vi "Dual Camera Delay Capture.vi"(7 "Calling VI Ref":refnum<vi>) -> ()   [LabVIEW 2016]
uses:
  Dual Camera Control Type Defs/Dual Camera Notifier Type.ctl
  Dual Camera Control Type Defs/Dual Camera Actions.ctl
  <vilib>/Utility/miscctls.llb/LVPointTypeDef.ctl
  Dual Camera Control Type Defs/Dual Camera Delay Capture Actions.ctl
panel:
  in  "Capture":bool
  out "Current Cycle":u32=1
  out "Current Delay Time (s)":dbl=1.0 format="%.1f"
  in  "Quit":bool
  in  "Cycle Delay (s)":u32
  in  "Number of Cycles":u32=1
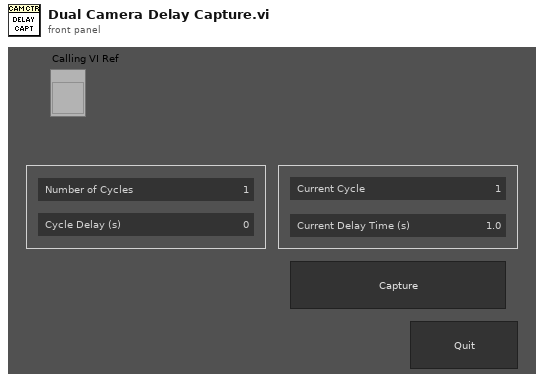
[diagram p1: front panel]
types:
  T1 = typedef "Dual Camera Delay Capture Actions.ctl" = enum16{"Idle", "Start Acquisition", "Get Images", "Check Cycle", "Delay", "Abort", "Exit Loop", "Quit"}
  T2 = enum16{"Always On", "Always Off", "Off While Running"}
  T3 = typedef "LVPointTypeDef.ctl" = cluster{"Horizontal":i16, "Vertical":i16}
  T4 = typedef "Dual Camera Notifier Type.ctl" = cluster{"Actions":T5, "Exposure Time (s)":dbl, "Num of Frames":u32, "Save Path":path, "Running?":bool, "Active Cameras":bool[]}
  T5 = typedef "Dual Camera Actions.ctl" = enum16{"Idle", "Exposure Time", "Preview", "Capture", "Set Save Path", "Lasers On", "Lasers Off", "Start Acquisition", "Abort", "Exit Loop", "Quit"}
  T6 = typedef "LVRectTypeDef.ctl" = cluster{"Left":i16, "Top":i16, "Right":i16, "Bottom":i16}
  T7 = typedef "LVBoundsTypeDef.ctl" = cluster{"Width":u32, "Height":u32}
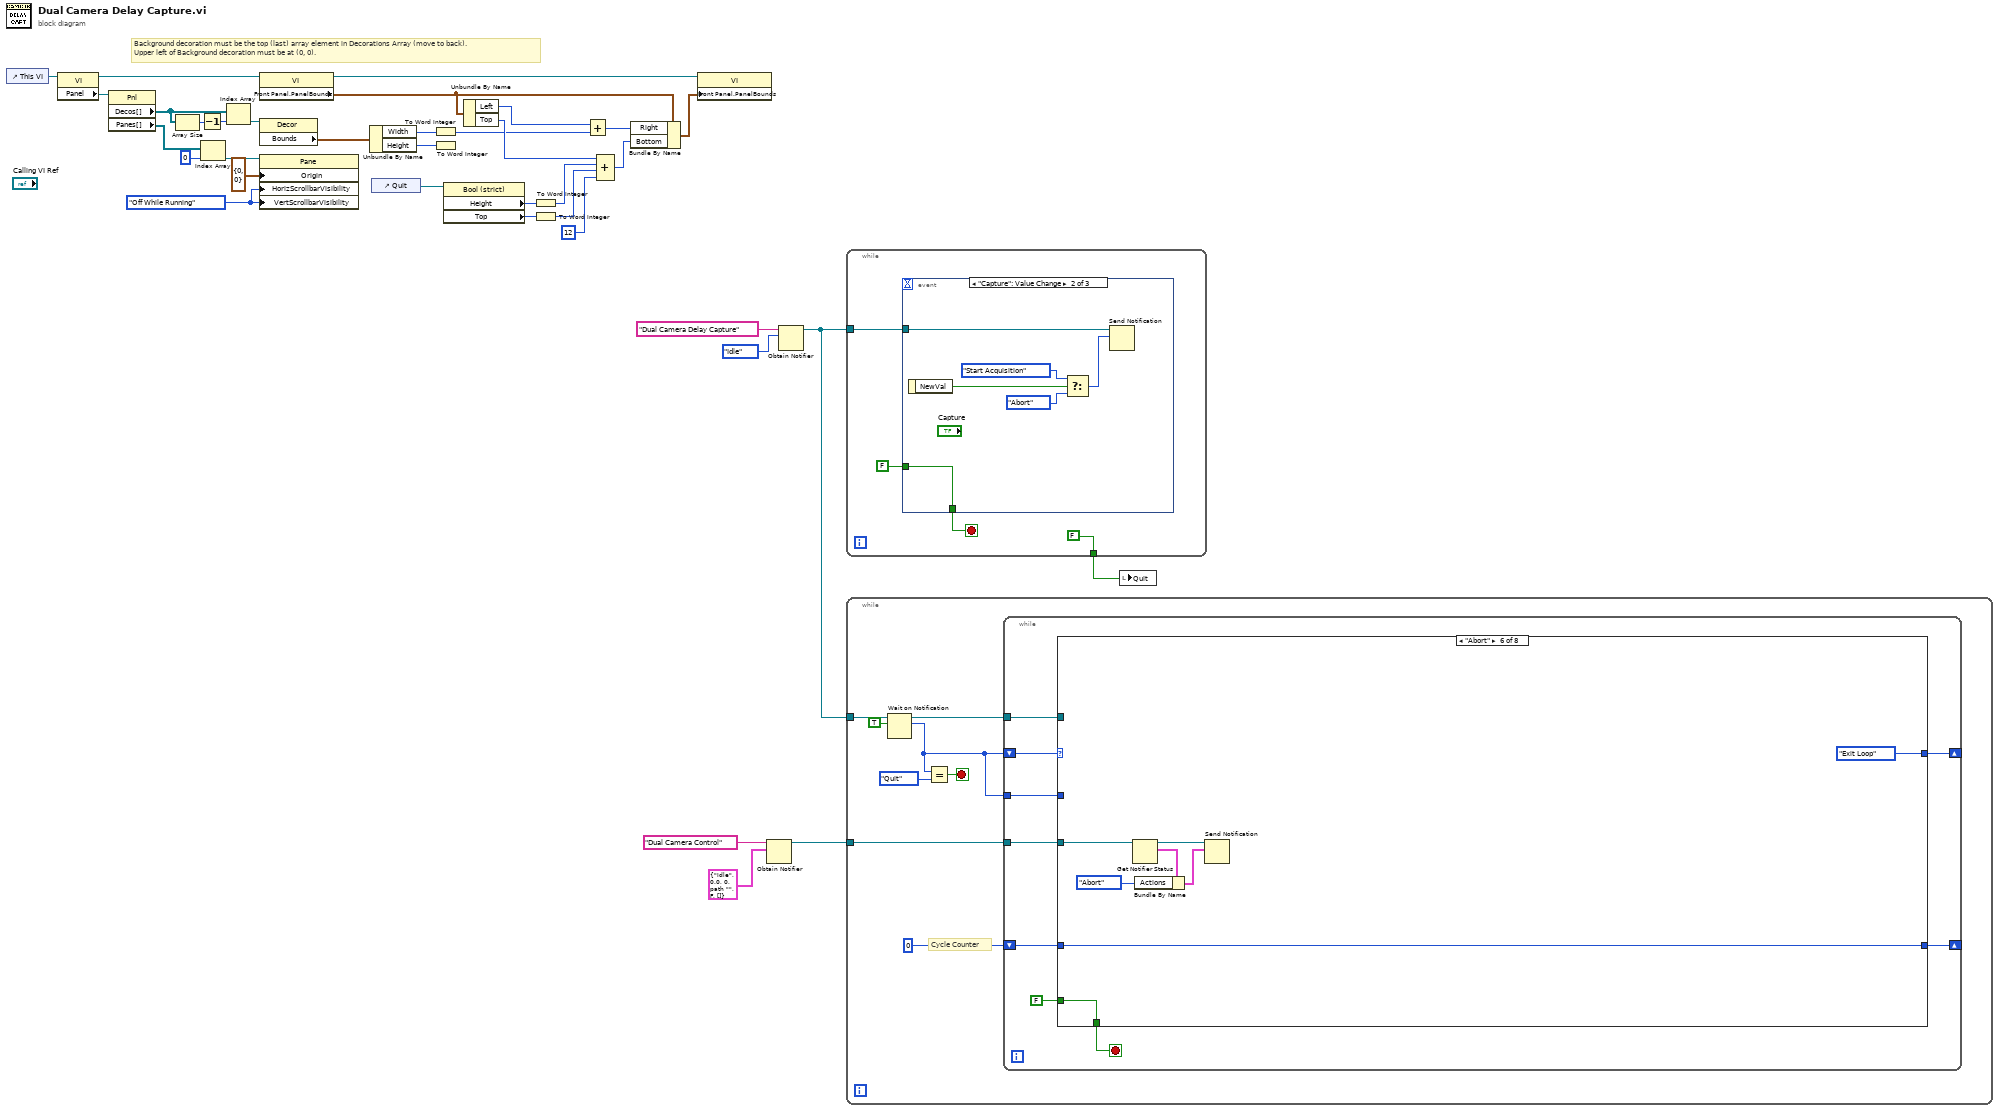
[diagram p0: block diagram]
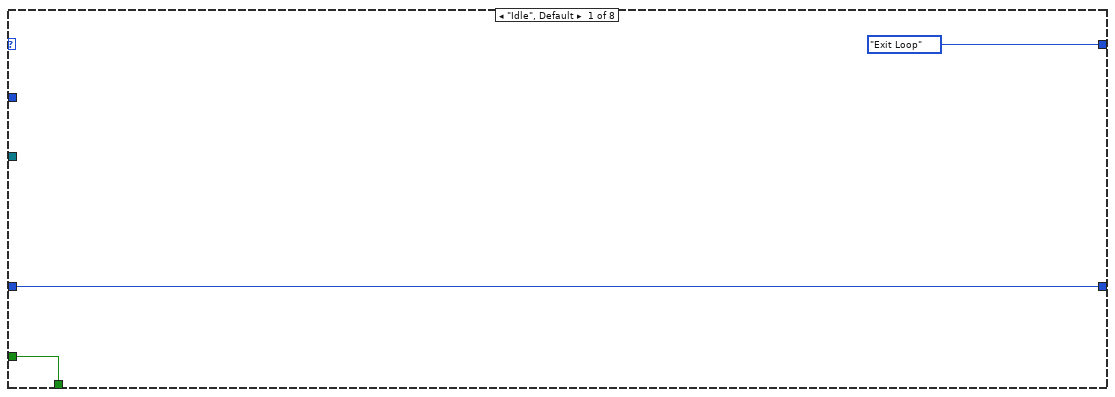
[diagram p2: hidden frame]
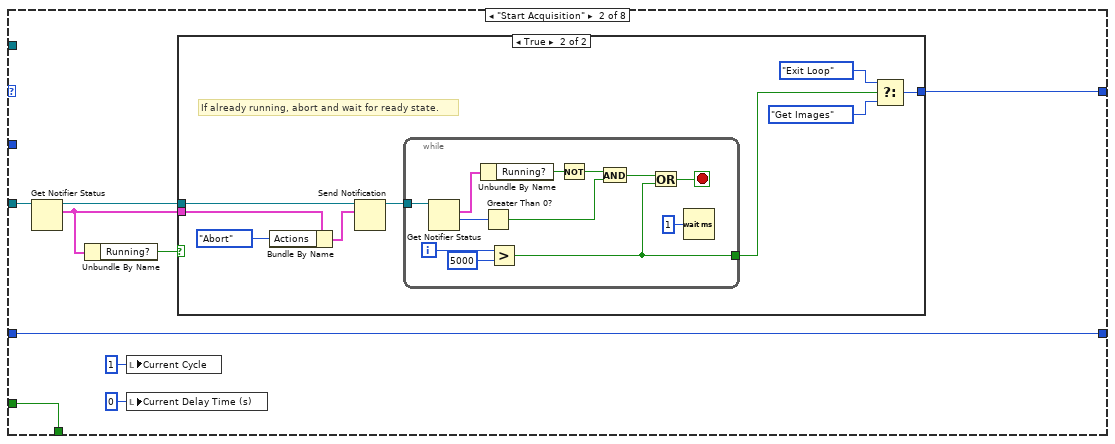
[diagram p3: hidden frame]
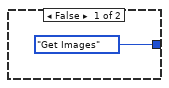
[diagram p4: hidden frame]
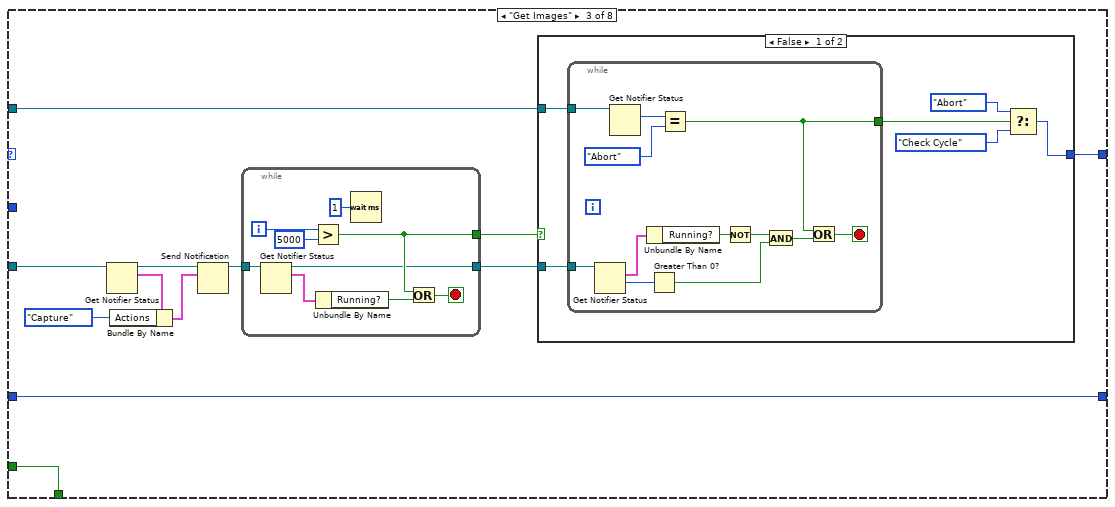
[diagram p5: hidden frame]
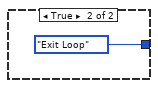
[diagram p6: hidden frame]
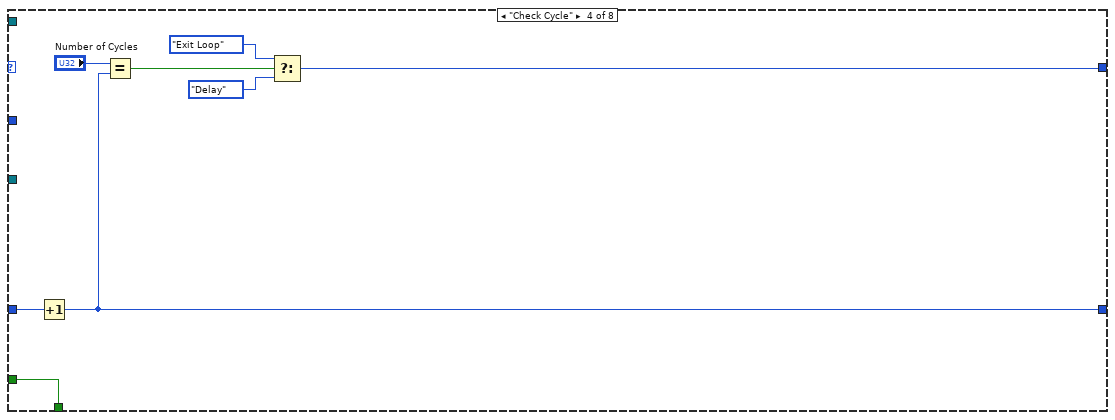
[diagram p7: hidden frame]
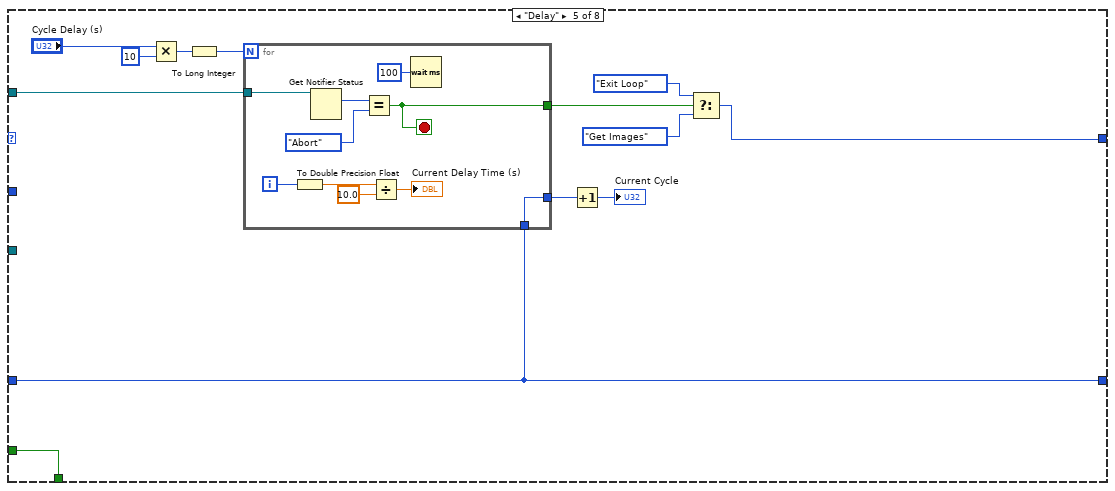
[diagram p8: hidden frame]
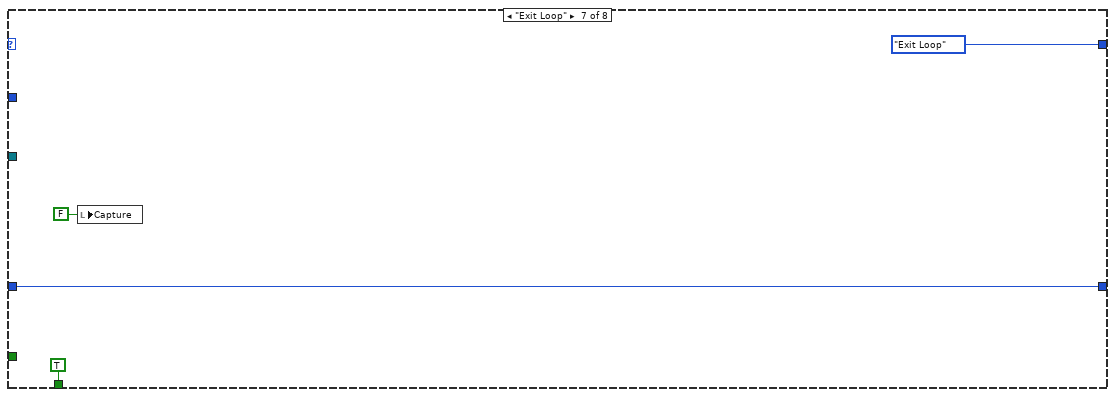
[diagram p9: hidden frame]
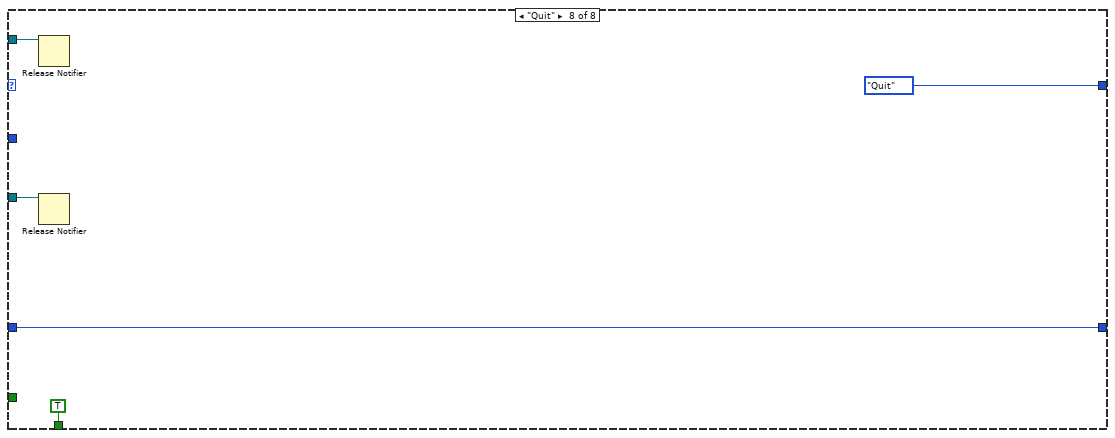
[diagram p10: hidden frame]
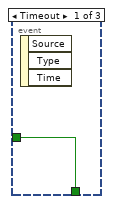
[diagram p11: hidden frame]
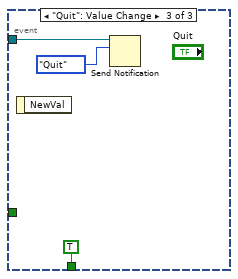
[diagram p12: hidden frame]
diagram:
  w17 = T2."Off While Running" ("Vertical Scrollbar Visibility")
  # "Background decoration must be the top (last) array element in Decorations Array (move to back).\nUpper left of Background decoration must be at (0, 0)."
  n1 = control-ref of="This VI"() -> (w9:refnum<vi>)
  n2 = property class="VI"(reference=w9) -> (reference out=w18:refnum<vi>, "Panel"=w10:refnum<vi>)  [unwired: 1 in, 1 out]
  n3 = property class="Pnl"(reference=w10) -> ("Decos[]"=w8:refnum<vi>[], "Panes[]"=w14:refnum<vi>[])  [unwired: 1 in, 2 out]
  n4 = Array Size(array=w8) -> (size(s)=w6:i32)
  n5 = Decrement(x=w6) -> (x-1=w7:i32)
  n6 = Index Array(array=w14, index=0) -> (element=w13:refnum<vi>)
  n7 = Index Array(array=w8, index=w7) -> (element=w16:refnum<vi>)
  n8 = property class="VI"(reference=w18) -> (reference out=w20:refnum<vi>, "Front Panel.PanelBounds"=w21:T6)  [unwired: 1 in, 1 out]
  n9 = property class="Decor"(reference=w16) -> ("Bounds"=w19:T7)  [unwired: 1 in, 2 out]
  n10 = property class="Pane"(reference=w13, "Origin"=T3 {"Horizontal"=0, "Vertical"=0}, "HorizScrollbarVisibility"=w17, "VertScrollbarVisibility"=w17) -> ()  [unwired: 1 in, 2 out]
  n11 = Unbundle By Name(w19) -> ("Width"=w24:u32, "Height"=w27:u32)
  n12 = control-ref of="Quit"() -> (w11:refnum<vi>)
  n13 = To Word Integer(number=w24) -> (16bit integer=w26:i16)
  n14 = To Word Integer(number=w27) -> ()  [unwired: 1 out]
  n15 = property class="Bool (strict)"(reference=w11) -> ("Height"=w29:u32, "Top"=w30:i32)  [unwired: 1 in, 2 out]
  n16 = Unbundle By Name(w21) -> ("Left"=w23:i16, "Top"=w34:i16)
  n17 = To Word Integer(number=w29) -> (16bit integer=w32:i16)
  n18 = To Word Integer(number=w30) -> (16bit integer=w33:i16)
  n19 = Add(x=w23, y=w26) -> (x+y=w25:i16)
  n20 = Compound Arithmetic op=ADD(w34, w32, w33, i16 12 ("y")) -> (w28:i16)
  n21 = Bundle By Name(cluster=w21, "Right"=w25, "Bottom"=w28) -> (w22:T6)
  n22 = property class="VI"(reference=w20, "Front Panel.PanelBounds"=w22) -> ()  [unwired: 1 in, 2 out]
  n23 = Obtain Notifier(name (unnamed)="Dual Camera Control", notification data type=T4 {"Actions"=enum."Idle", "Exposure Time (s)"=0.0, "Num of Frames"=0, "Save Path"=path "", "Running?"=FALSE, "Active Cameras"=[]} ("Dual Camera Notifier Type")) -> (notifier out=w4:refnum<notifier>)  [unwired: 2 in, 2 out]
  n24 = Obtain Notifier(name (unnamed)="Dual Camera Delay Capture", notification data type=Dual_Camera_Delay_Capture_Actions."Idle" ("Actions")) -> (notifier out=w1:refnum<notifier>)  [unwired: 2 in, 2 out]
  n25 = while {
    tunnel: [FALSE] -> w35
    tunnel: w1 -> [w37]
    stop <- w39 stop-if-true
    n26 = event shown="[1] \"Capture\": Value Change" {
      selector: _ -> [_ _ _]
      dyn-events: _ -> [_ _ _]
      timeout: _ -> [_ _ _]
      tunnel: FALSE -> [w41 w47 _]
      tunnel: [w41 w47 TRUE] -> w39
      tunnel: w37 -> [_ w43 w49]
      event Timeout {
        n27 = event-data() -> ()  [unwired: 1 in, 3 out]
      }
      event "Capture": Value Change {
        n28 = event-data() -> ("NewVal"=w46:bool)  [unwired: 1 in]
        n29 = Select(t=Dual_Camera_Delay_Capture_Actions."Start Acquisition" ("notification"), s=w46, f=Dual_Camera_Delay_Capture_Actions."Abort" ("notification")) -> (s? t:f=w42:T1)
        n30 = Send Notification(notification=w42, notifier=w43) -> ()  [unwired: 1 in, 2 out]
      }
      event "Quit": Value Change {
        n31 = event-data() -> ()  [unwired: 1 in, 1 out]
        n32 = Send Notification(notification=Dual_Camera_Delay_Capture_Actions."Quit", notifier=w49) -> ()  [unwired: 1 in, 2 out]
      }
    }
  }
  n33 = while {
    tunnel: w1 -> [w58]
    tunnel: w4 -> [w54]
    stop <- w56 stop-if-true
    # "Cycle Counter"
    n34 = Wait on Notification(notifier=w58, ignore previous (F)=TRUE) -> (notifier out=w55:refnum<notifier>, notification=w53:T1)  [unwired: 2 in, 2 out]
    n35 = Equal?(x=w53, y=Dual_Camera_Delay_Capture_Actions."Quit") -> (x = y?=w56:bool)
    n36 = while {
      shift-right: [w61] -> _
      shift-left: w53 -> [w66]
      tunnel: w55 -> [w67]
      tunnel: w53 -> [w63]
      tunnel: w54 -> [w62]
      shift-right: [w59] -> _
      shift-left: u32 0 -> [w60]
      stop <- w64 stop-if-true
      n37 = case shown="\"Abort\"" w66 {
        tunnel: w67 -> [_ _ w106 _ w157 _ _ w189]
        tunnel: FALSE -> [w70 w79 w113 w149 w162 w180 _ _]
        tunnel: [w70 w79 w113 w149 w162 w180 TRUE TRUE] -> w64
        tunnel: w63 -> [_ _ _ _ _ _ _ _]
        tunnel: w62 -> [_ w75 w109 _ _ w173 _ w185]
        tunnel: [Dual_Camera_Delay_Capture_Actions."Exit Loop" ("y") w71 w105 w142 w153 Dual_Camera_Delay_Capture_Actions."Exit Loop" ("y") Dual_Camera_Delay_Capture_Actions."Exit Loop" ("y") Dual_Camera_Delay_Capture_Actions."Quit" ("y")] -> w61
        tunnel: w60 -> [w69 w78 w112 w148 w152 w179 w183 w186]
        tunnel: [w69 w78 w112 w147 w152 w179 w183 w186] -> w59
        frame "Idle", Default {
        }
        frame "Start Acquisition" {
          n38 = Get Notifier Status(notifier=w75) -> (notifier out=w73:refnum<notifier>, current notification=w72:T4)  [unwired: 1 in, 3 out]
          n39 = Unbundle By Name(w72) -> ("Running?"=w74:bool)
          n40 = local write "Current Cycle"(u32 1 ("Current Cycle")) -> ()
          n41 = local write "Current Delay Time (s)"(u32 0 ("Current Delay Time (s)")) -> ()
          n42 = case shown="True" w74 {
            tunnel: w73 -> [_ w88]
            tunnel: w72 -> [_ w87]
            tunnel: [Dual_Camera_Delay_Capture_Actions."Get Images" ("y") w81] -> w71
            frame False {
            }
            frame True {
              # "If already running, abort and wait for ready state."
              n43 = Bundle By Name(cluster=w87, "Actions"=Dual_Camera_Actions."Abort") -> (w89:T4)
              n44 = Send Notification(notification=w89, notifier=w88) -> (notifier out=w85:refnum<notifier>)  [unwired: 1 in, 1 out]
              n45 = while {
                tunnel: w85 -> [w101]
                tunnel: [w90] -> w82
                i -> [w93]
                stop <- w91 stop-if-true
                n46 = Get Notifier Status(notifier=w101) -> (current notification=w100:T4, # waiting=w98:i32)  [unwired: 1 in, 3 out]
                n47 = Unbundle By Name(w100) -> ("Running?"=w99:bool)
                n48 = Greater Than 0?(x=w98) -> (x > 0?=w96:bool)
                n49 = Greater?(x=w93, y=5000) -> (0:w90:bool)
                n50 = Not(x=w99) -> (.not. x?=w97:bool)
                n51 = And(x=w97, y=w96) -> (x .and. y?=w95:bool)
                n52 = Or(x=w95, y=w90) -> (x .or. y?=w91:bool)
                n53 = Wait (ms)(milliseconds to wait=u32 1) -> ()  [unwired: 1 out]
              }
              n54 = Select(t=Dual_Camera_Delay_Capture_Actions."Exit Loop" ("y"), s=w82, f=Dual_Camera_Delay_Capture_Actions."Get Images" ("y")) -> (s? t:f=w81:T1)
            }
          }
        }
        frame "Get Images" {
          n55 = Get Notifier Status(notifier=w109) -> (notifier out=w108:refnum<notifier>, current notification=w107:T4)  [unwired: 1 in, 3 out]
          n56 = Bundle By Name(cluster=w107, "Actions"=Dual_Camera_Actions."Capture") -> (w111:T4)
          n57 = Send Notification(notification=w111, notifier=w108) -> (notifier out=w104:refnum<notifier>)  [unwired: 1 in, 1 out]
          n58 = while {
            tunnel: w104 -> [w122]
            tunnel: [w115] -> w103
            tunnel: [w114] -> w102
            i -> [w117]
            stop <- w119 stop-if-true
            n59 = Get Notifier Status(notifier=w122) -> (notifier out=w114:refnum<notifier>, current notification=w121:T4)  [unwired: 1 in, 3 out]
            n60 = Greater?(x=w117, y=5000) -> (0:w115:bool)
            n61 = Unbundle By Name(w121) -> ("Running?"=w120:bool)
            n62 = Wait (ms)(milliseconds to wait=u32 1) -> ()  [unwired: 1 out]
            n63 = Or(x=w115, y=w120) -> (x .or. y?=w119:bool)
          }
          n64 = case shown="False" w103 {
            tunnel: w102 -> [w128 _]
            tunnel: w106 -> [w127 _]
            tunnel: [w123 Dual_Camera_Delay_Capture_Actions."Exit Loop" ("y")] -> w105
            frame False {
              n65 = while {
                tunnel: w128 -> [w140]
                tunnel: w127 -> [w133]
                tunnel: [w129] -> w126
                stop <- w134 stop-if-true
                n66 = Get Notifier Status(notifier=w140) -> (current notification=w139:T4, # waiting=w137:i32)  [unwired: 1 in, 3 out]
                n67 = Get Notifier Status(notifier=w133) -> (current notification=w131:T1)  [unwired: 1 in, 4 out]
                n68 = Unbundle By Name(w139) -> ("Running?"=w138:bool)
                n69 = Greater Than 0?(x=w137) -> (x > 0?=w135:bool)
                n70 = Equal?(x=w131, y=Dual_Camera_Delay_Capture_Actions."Abort") -> (x = y?=w129:bool)
                n71 = Not(x=w138) -> (.not. x?=w136:bool)
                n72 = And(x=w136, y=w135) -> (x .and. y?=w132:bool)
                n73 = Or(x=w129, y=w132) -> (x .or. y?=w134:bool)
              }
              n74 = Select(t=Dual_Camera_Delay_Capture_Actions."Abort" ("y"), s=w126, f=Dual_Camera_Delay_Capture_Actions."Check Cycle" ("y")) -> (s? t:f=w123:T1)
            }
            frame True {
            }
          }
        }
        frame "Check Cycle" {
          n75 = Increment(x=w148) -> (x+1=w147:u32)
          n76 = Equal?(x="Number of Cycles", y=w147) -> (x = y?=w145:bool)
          n77 = Select(t=Dual_Camera_Delay_Capture_Actions."Exit Loop" ("y"), s=w145, f=Dual_Camera_Delay_Capture_Actions."Delay" ("y")) -> (s? t:f=w142:T1)
        }
        frame "Delay" {
          n78 = Multiply(x="Cycle Delay (s)", y=u32 10) -> (x*y=w159:u32)
          n79 = To Long Integer(number=w159) -> (32bit integer=w158:i32)
          n80 = for {
            N: w158 -> [_]
            tunnel: w157 -> [w171]
            tunnel: [w168] -> w156
            tunnel: w152 -> [w163]
            tunnel: [w163] -> w150
            i -> [w167]
            stop <- w168 stop-if-true
            n81 = To Double Precision Float(number=w167) -> (double precision float=w166:dbl)
            n82 = Get Notifier Status(notifier=w171) -> (current notification=w170:T1)  [unwired: 1 in, 4 out]
            n83 = Equal?(x=w170, y=Dual_Camera_Delay_Capture_Actions."Abort") -> (x = y?=w168:bool)
            n84 = Divide(x=w166, y=10.0) -> (x/y=→"Current Delay Time (s)":dbl)
            n85 = Wait (ms)(milliseconds to wait=u32 100) -> ()  [unwired: 1 out]
          }
          n86 = Increment(x=w150) -> (x+1=→"Current Cycle":u32)
          n87 = Select(t=Dual_Camera_Delay_Capture_Actions."Exit Loop" ("y"), s=w156, f=Dual_Camera_Delay_Capture_Actions."Get Images" ("y")) -> (s? t:f=w153:T1)
        }
        frame "Abort" {
          n88 = Get Notifier Status(notifier=w173) -> (notifier out=w175:refnum<notifier>, current notification=w174:T4)  [unwired: 1 in, 3 out]
          n89 = Bundle By Name(cluster=w174, "Actions"=Dual_Camera_Actions."Abort") -> (w177:T4)
          n90 = Send Notification(notification=w177, notifier=w175) -> ()  [unwired: 1 in, 2 out]
        }
        frame "Exit Loop" {
          n91 = local write "Capture"(FALSE ("Capture")) -> ()
        }
        frame "Quit" {
          n92 = Release Notifier(notifier=w189) -> ()  [unwired: 2 in, 3 out]
          n93 = Release Notifier(notifier=w185) -> ()  [unwired: 2 in, 3 out]
        }
      }
    }
  }
  n94 = local write "Quit"(w35) -> ()
